vi "Autonomous Independent.vi"   [LabVIEW 2012]
doc: "This VI is called when autonomous begins, and will automatically be terminated when autonomous ends. You can carry out timed or sensor driven robot movement independently without needing to return to the caller."
uses:
  <vilib>/Rock Robotics/WPI/Relay/WPI_RelayValue.ctl
  Robot Global Data.vi
types:
  T1 = typedef "WPI_EncoderDevRef.ctl" = cluster{"DevStatus":errorcluster, "EncoderIndex":T2, "CounterIndex":T3, "DistancePerCount":dbl, "Decoding Type":T4}
  T2 = typedef "FPGA_EncoderIdx.ctl" = enum8{"Enc 0", "Enc 1", "Enc 2", "Enc 3", "Invalid"}
  T3 = typedef "FPGA_CounterCtrSystemIndex.ctl" = enum8{"Ctr 0", "Ctr 1", "Ctr 2", "Ctr 3", "Ctr 4", "Ctr 5", "Ctr 6", "Ctr 7", "Invalid"}
  T4 = typedef "WPI_EncoderType.ctl" = enum16{"1x", "2x", "4x"}
  T5 = typedef "WPI_GyroDevRef.ctl" = cluster{"DevStatus":errorcluster, "Analog Module":T6, "Analog Channel":T7, "Offset":dbl, "Gain (VoltsPerDegree/Second)":dbl}
  T6 = typedef "FPGA_TypedefAnalogModule.ctl" = enum16{"Analog Module 1", "Analog Module 2"}
  T7 = typedef "FPGA_AIChannel.ctl" = enum8{"AI 1", "AI 2", "AI 3", "AI 4", "AI 5", "AI 6", "AI 7", "AI 8", "Invalid"}
  T8 = typedef "WPI_MotorControlDeviceRef.ctl" = cluster{"DeviceStatus":errorcluster, "Type":enum16{"PWM", "CAN"}, "PWM":cluster{"Digital Module":T9, "PWM Channel":T10, "DeadBand":T11}, "CAN":cluster{"Device Number":u8, "Control Mode":T12, "Semaphore":T13, "Max Vout":dbl}, "Invert":bool, "TransformRef":T14, "InvTransformRef":T14}
  T9 = typedef "FPGA_TypedefDigitalModule.ctl" = enum16{"Digital Module 1", "Digital Module 2"}
  T10 = typedef "FPGA_DIOPWMChannel.ctl" = enum8{"PWM 1", "PWM 2", "PWM 3", "PWM 4", "PWM 5", "PWM 6", "PWM 7", "PWM 8", "PWM 9", "PWM 10", "Invalid"}
  T11 = typedef "WPI_PWMDeadband.ctl" = cluster{"Name":string, "maxPositivePwm":i32, "minPositivePwm":i32, "centerPwm":i32, "maxNegativePwm":i32, "minNegativePwm":i32, "angularRange":u16}
  T12 = typedef "WPI_CANJaguar_ControlMode.ctl" = enum8{"Percent VBus", "Current", "Speed", "Position", "Voltage"}
  T13 = typedef "Semaphore RefNum" = refnum<k1>
  T14 = typedef "WPI_PWMTransform_ConPane.ctl" = refnum<vi>
  T15 = typedef "WPI_RelayValue.ctl" = enum16{"Off", "On", "Forward", "Reverse"}
  T16 = typedef "WPI_DigitalInputDevRef.ctl" = cluster{"DevStatus":errorcluster, "DIO Channel":T17, "Digital Module":T9}
  T17 = typedef "FPGA_DIOChannel.ctl" = enum8{"DIO 1", "DIO 2", "DIO 3", "DIO 4", "DIO 5", "DIO 6", "DIO 7", "DIO 8", "DIO 9", "DIO 10", "DIO 11", "DIO 12", "DIO 13", "DIO 14", "Invalid"}
  T18 = typedef "WPI_RelayDevRef.ctl" = cluster{"DevStatus":errorcluster, "Relay Channel":T19, "Digital Module":T9, "Relay Direction":T20}
  T19 = typedef "FPGA_DIORelayChannel.ctl" = enum8{"Relay 1", "Relay 2", "Relay 3", "Relay 4", "Relay 5", "Relay 6", "Relay 7", "Relay 8", "Invalid"}
  T20 = typedef "WPI_RelayDirection.ctl" = enum16{"Both directions", "Forward only", "Reverse only"}
  T21 = cluster{"Right Servo High":dbl, "Right Servo Mid":dbl, "Right Servo Low":dbl, "Left Servo High":dbl, "Left Servo Mid":dbl, "Left Servo Low":dbl}
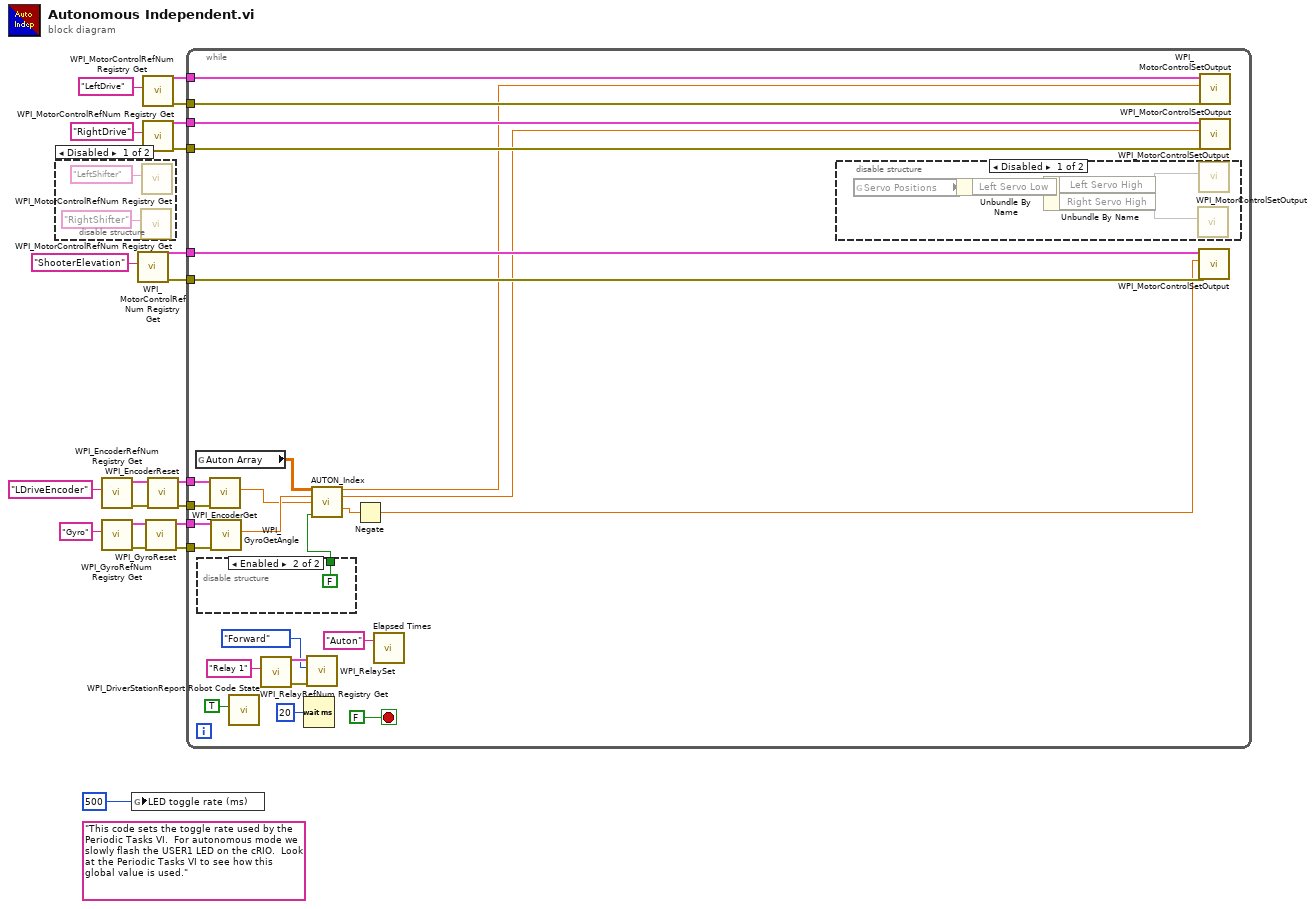
[diagram p0: block diagram]
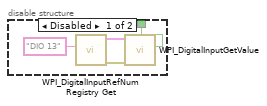
[diagram p3: hidden frame]
diagram:
  (unwired) "This code sets the toggle rate used by the Periodic Tasks VI.  For autonomous mode we slowly flash the USER1 LED on the cRIO.  Look at the Periodic Tasks VI to see how this global value is used."
  n1 = disable-structure shown="Disabled" {
    frame Disabled {
      n2 = call <vilib>:"WPI_MotorControlRefNum Registry Get.vi"("refnum name"="RightShifter") -> ()  [unwired: 9 in, 2 out]
      n3 = call <vilib>:"WPI_MotorControlRefNum Registry Get.vi"("refnum name"="LeftShifter") -> ()  [unwired: 9 in, 2 out]
    }
    frame Enabled {
    }
  }
  n4 = call <vilib>:"WPI_EncoderRefNum Registry Get.vi"("refnum name"="LDriveEncoder") -> ("error out"=w4:errorcluster, "EncoderDevRef"=w3:T1)  [unwired: 9 in]
  n5 = call <vilib>:"WPI_GyroRefNum Registry Get.vi"("refnum name"="Gyro") -> ("error out"=w8:errorcluster, "GyroDevRef"=w9:T5)  [unwired: 9 in]
  n6 = global write "Robot Global Data.vi" "LED toggle rate (ms)"(u32 500 ("LED ms toggle rate")) -> ()
  n7 = call <vilib>:"WPI_MotorControlRefNum Registry Get.vi"("refnum name"="ShooterElevation") -> ("error out"=w11:errorcluster, "MotorControlDevRef"=w12:T8)  [unwired: 9 in]
  n8 = call <vilib>:"WPI_MotorControlRefNum Registry Get.vi"("refnum name"="LeftDrive") -> ("error out"=w17:errorcluster, "MotorControlDevRef"=w18:T8)  [unwired: 9 in]
  n9 = call <vilib>:"WPI_MotorControlRefNum Registry Get.vi"("refnum name"="RightDrive") -> ("error out"=w16:errorcluster, "MotorControlDevRef"=w15:T8)  [unwired: 9 in]
  n10 = call <vilib>:"WPI_GyroReset.vi"("error in (no error)"=w8, "GyroDevRef"=w9) -> ("error out"=w6:errorcluster, "GyroDevRef"=w7:T5)  [unwired: 8 in]
  n11 = call <vilib>:"WPI_EncoderReset.vi"("error in (no error)"=w4, "EncoderDevRef"=w3) -> ("error out"=w1:errorcluster, "EncoderDevRef"=w2:T1)  [unwired: 8 in]
  n12 = while {
    tunnel: w18 -> [w45]
    tunnel: w17 -> [w44]
    tunnel: w15 -> [w42]
    tunnel: w16 -> [w43]
    tunnel: w12 -> [w39]
    tunnel: w11 -> [w38]
    tunnel: w7 -> [w33]
    tunnel: w6 -> [w32]
    tunnel: w2 -> [w31]
    tunnel: w1 -> [w30]
    stop <- FALSE stop-if-true
    n13 = global read "Robot Global Data.vi" "Auton Array"() -> (w41:dbl[][])
    n14 = disable-structure shown="Enabled" {
      disable-tunnel: [w52 FALSE ("Harvester DIO")] -> w23
      frame Disabled {
        n15 = call <vilib>:"WPI_DigitalInputRefNum Registry Get.vi"("refnum name"="DIO 13") -> ("error out"=w49:errorcluster, "DigitalInputDevRef"=w50:T16)  [unwired: 9 in]
        n16 = call <vilib>:"WPI_DigitalInputGetValue.vi"("error in (no error)"=w49, "DigitalInputDevRef"=w50) -> ("Value"=w52:bool)  [unwired: 7 in, 2 out]
      }
      frame Enabled {
      }
    }
    n17 = call <vilib>:"WPI_EncoderGet.vi"("error in (no error)"=w30, "EncoderDevRef"=w31) -> ("Distance"=w29:dbl)  [unwired: 4 in, 5 out]
    n18 = call <vilib>:"WPI_GyroGetAngle.vi"("error in (no error)"=w32, "GyroDevRef"=w33) -> ("Angle"=w40:dbl)  [unwired: 6 in, 3 out]
    n19 = call <vilib>:"WPI_DriverStationReport Robot Code State.vi"("Autonomous"=TRUE) -> ()  [unwired: 10 in, 1 out]
    n20 = call <vilib>:"WPI_RelayRefNum Registry Get.vi"("refnum name"="Relay 1") -> ("error out"=w25:errorcluster, "RelayDevRef"=w27:T18)  [unwired: 9 in]
    n21 = Wait (ms)(milliseconds to wait=u32 20) -> ()  [unwired: 1 out]
    n22 = call <vilib>:"WPI_RelaySet.vi"("error in (no error)"=w25, "RelayValue"=WPI_RelayValue."Forward", "RelayDevRef"=w27) -> ()  [unwired: 7 in, 2 out]
    n23 = call "AUTON_Index.vi"("Auton Array"=w41, "MeasuredHeading"=w40, "LeftEncoder"=w29, "Harvester DIO"=w23) -> ("Left Drive"=w34:dbl, "Right Drive"=w35:dbl, "Shooter Elevation"=w37:dbl)  [unwired: 5 in, 4 out]
    n24 = Negate(x=w37) -> (-x=w36:dbl)
    n25 = call "Elapsed Times.vi"("Call Name"="Auton") -> ()  [unwired: 2 in, 1 out]
    n26 = disable-structure shown="Disabled" {
      frame Disabled {
        n27 = global read "Robot Global Data.vi" "Servo Positions"() -> (w57:T21)
        n28 = Unbundle By Name(w57) -> ("Left Servo Low"=w56:dbl)
        n29 = Unbundle By Name(w56) -> ("Left Servo High"=w55, "Right Servo High"=w54)
        n30 = call <vilib>:"WPI_MotorControlSetOutput.vi"("Output"=w54) -> ()  [unwired: 8 in, 3 out]
        n31 = call <vilib>:"WPI_MotorControlSetOutput.vi"("Output"=w55) -> ()  [unwired: 8 in, 3 out]
      }
      frame Enabled {
      }
    }
    n32 = call <vilib>:"WPI_MotorControlSetOutput.vi"("error in (no error)"=w38, "Output"=w36, "MotorControlDevRef"=w39) -> ()  [unwired: 6 in, 3 out]
    n33 = call <vilib>:"WPI_MotorControlSetOutput.vi"("error in (no error)"=w44, "Output"=w34, "MotorControlDevRef"=w45) -> ()  [unwired: 6 in, 3 out]
    n34 = call <vilib>:"WPI_MotorControlSetOutput.vi"("error in (no error)"=w43, "Output"=w35, "MotorControlDevRef"=w42) -> ()  [unwired: 6 in, 3 out]
  }
